vi "LC-MISDK_Meas_sub.vi"(0 ".NET refnum入力":refnum<k24>, 1 "Get Measurement Data":T1(radio)=enum."Lvxy", 8 "COM":i32) -> (10 "Duv":dbl, 12 "ReadLatestData Error":dbl format="%#_6f", 13 "Tcp":dbl, 14 "Lv 4":dbl, 15 "x":dbl, 16 "Z":dbl, 17 "Y":dbl, 18 "Lv 3":dbl, 19 "Dw":dbl, 20 "y":dbl, 21 "Lv":dbl, 22 "Pe":dbl, 23 "X":dbl, 24 "vd":dbl, 25 "Lv 2":dbl, 26 "ud":dbl)   [LabVIEW 2019]
uses:
  C:/Program Files (x86)/National Instruments/LabVIEW 2019/LC-MISDK.dll
  Program Files (x86)/National Instruments/LabVIEW 2019/LC-MISDK.dll
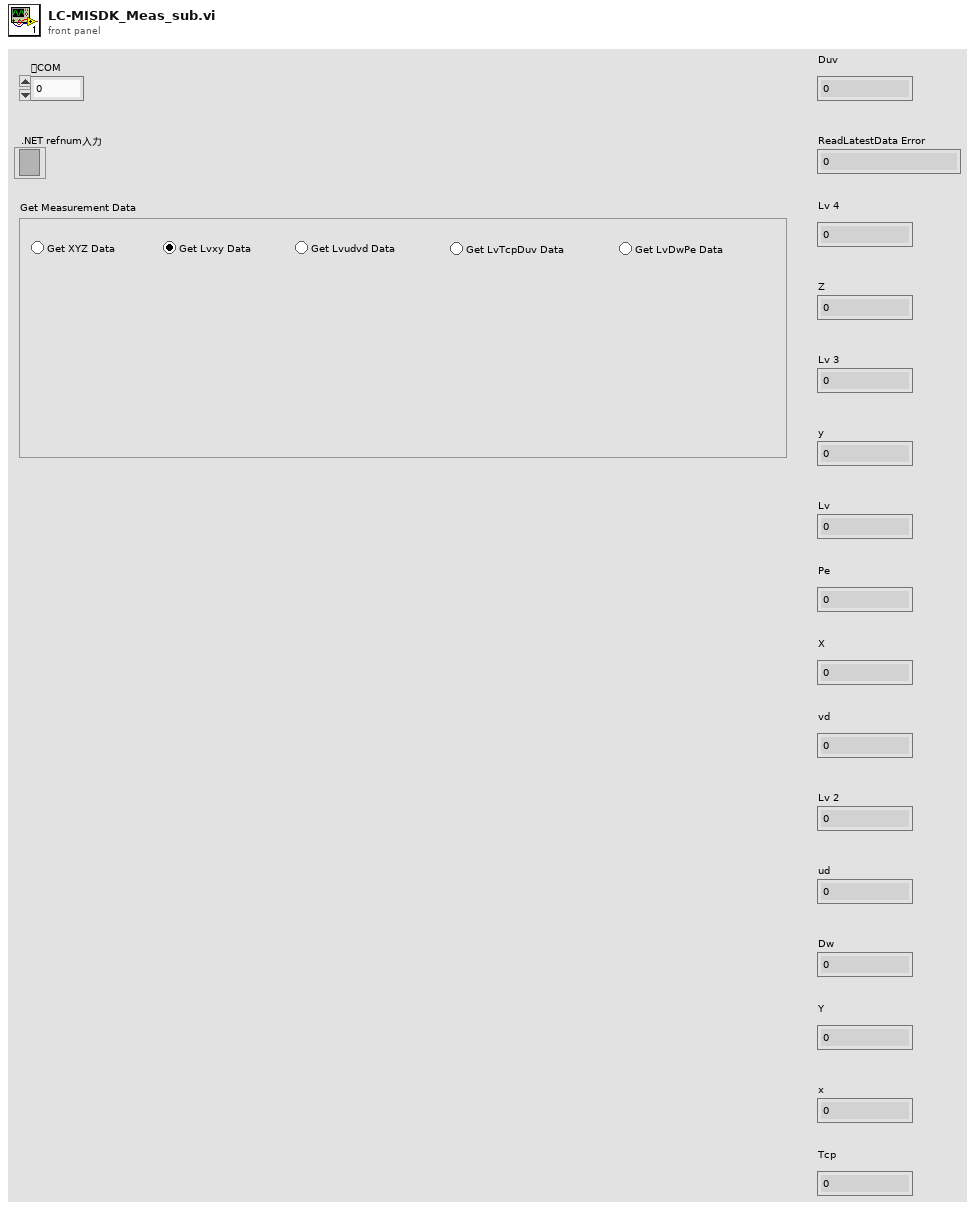
[diagram p1: front panel]
types:
  T1 = enum32{"XYZ", "Lvxy", "Lvudvd", "LvTcpDuv", "LvDwPe"}
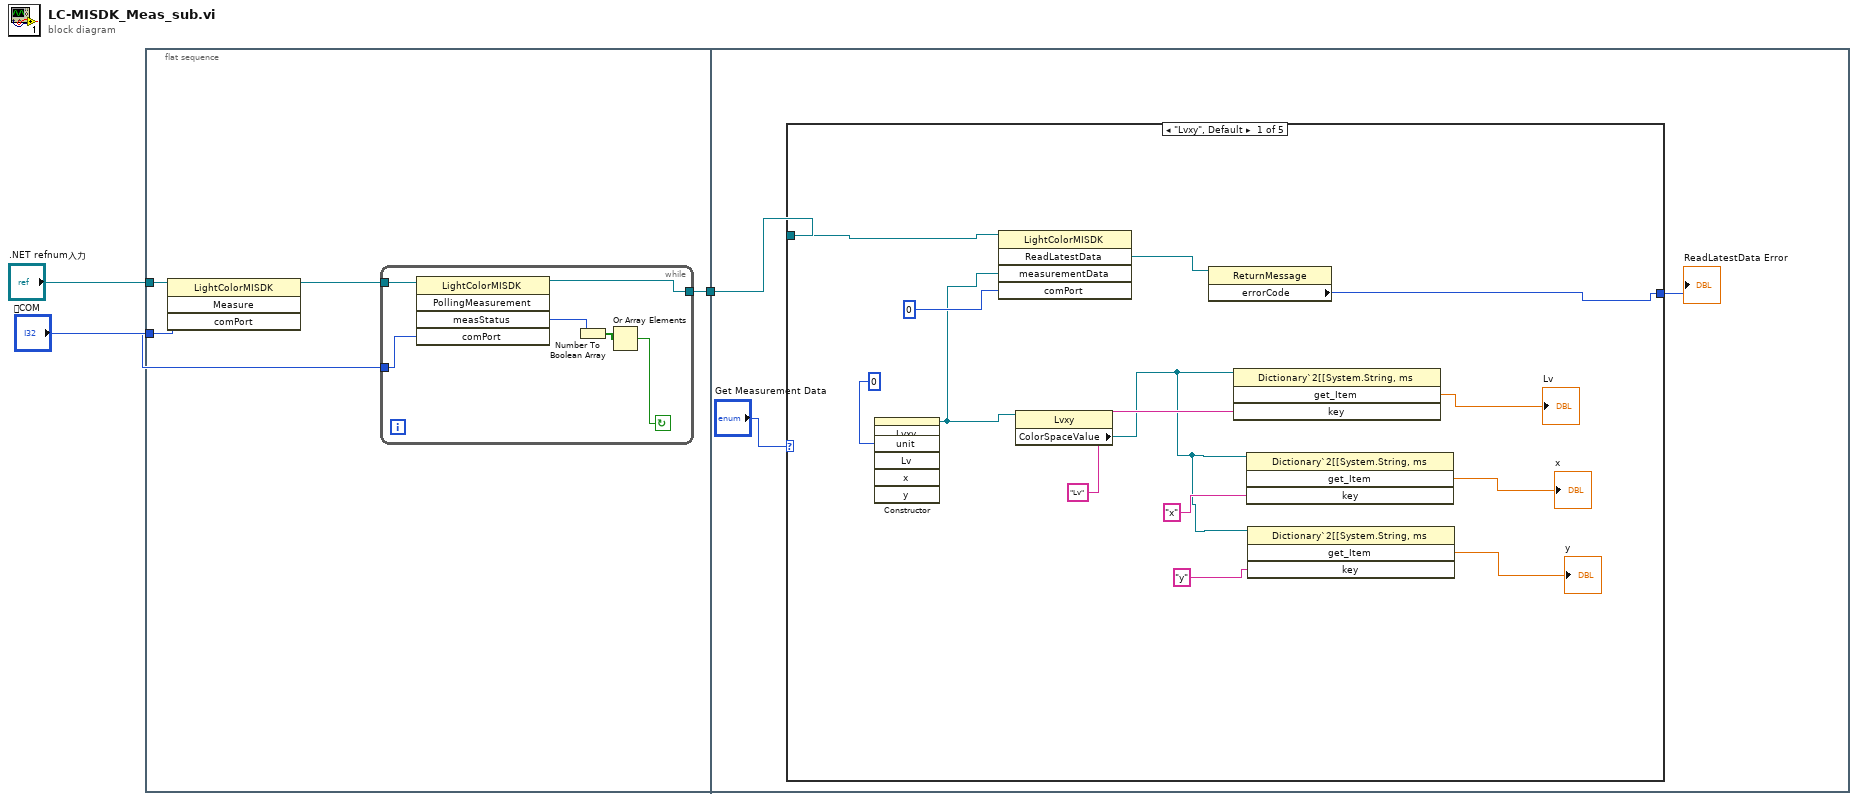
[diagram p0: block diagram]
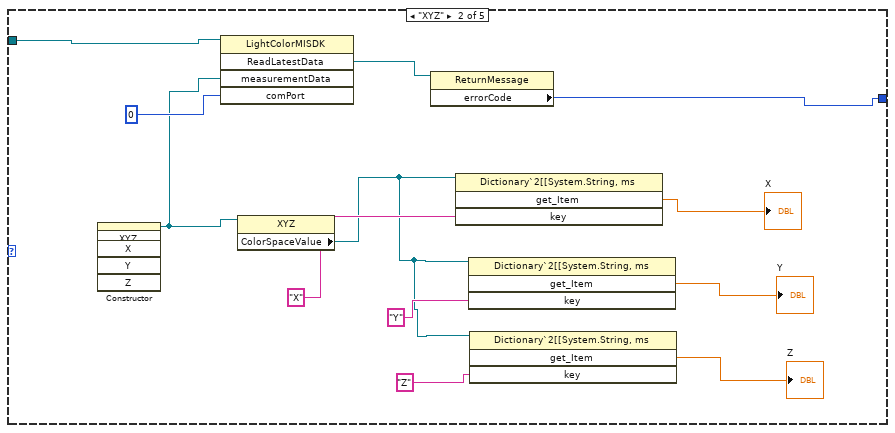
[diagram p2: hidden frame]
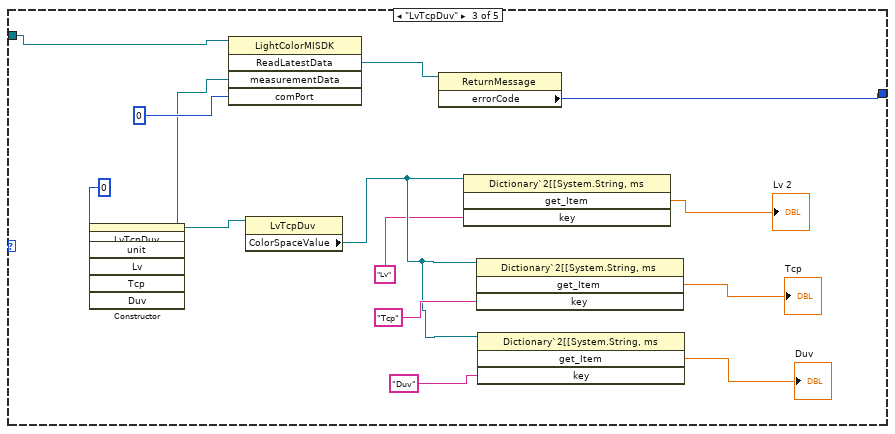
[diagram p3: hidden frame]
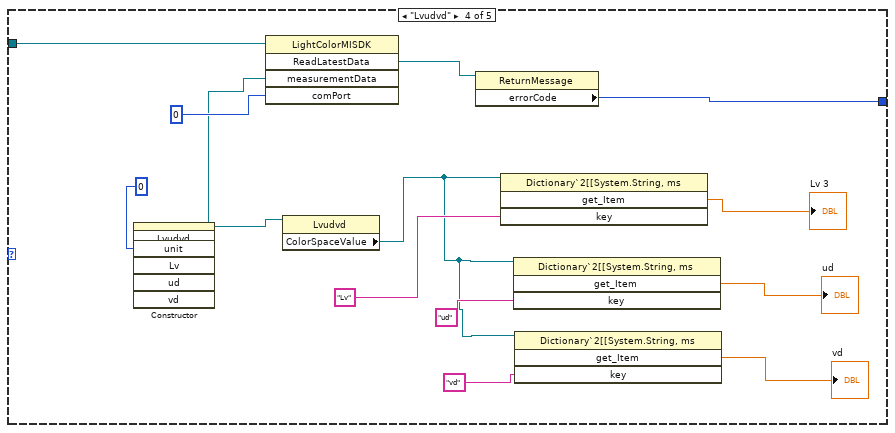
[diagram p4: hidden frame]
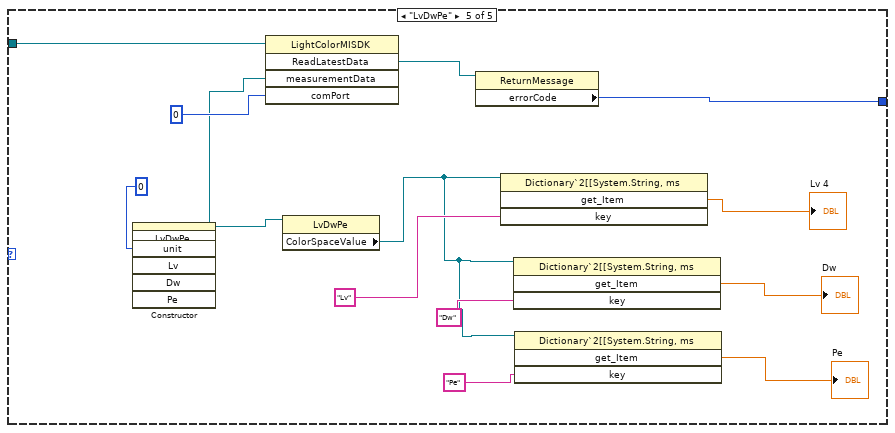
[diagram p5: hidden frame]
diagram:
  n1 = flat-sequence {
    tunnel: ".NET refnum入力" -> [w6]
    tunnel: "COM" -> [w4]
    tunnel: [w7] -> w3
    tunnel: w3 -> [w15]
    frame #0 {
      n2 = invoke on="インボークノード" class="LightColorMISDK" method="Measure"(reference=w6, "comPort"=w4) -> (reference out=w5:refnum<k24>)  [unwired: 2 in, 3 out]
      n3 = while {
        tunnel: [w12] -> w7
        tunnel: w5 -> [w11]
        tunnel: w4 -> [w10]
        stop <- w8 continue-if-true
        n4 = invoke on="インボークノード" class="LightColorMISDK" method="PollingMeasurement"(reference=w11, "comPort"=w10) -> (reference out=w12:refnum<k24>, "measStatus"=w13:i32)  [unwired: 3 in, 3 out]
        n5 = Number To Boolean Array(number=w13) -> (Boolean array=w9:bool[])
        n6 = Or Array Elements(Boolean array=w9) -> (logical OR=w8:bool)
      }
    }
    frame #1 {
      n7 = case shown="\"Lvxy\", Default" "Get Measurement Data" {
        tunnel: w15 -> [w29 w41 w54 w67 w80]
        tunnel: [w17 w30 w42 w55 w68] -> w14
        frame "Lvxy", Default {
          n8 = constructor class="Lvxy"("unit"=0) -> (reference out=w26:refnum<k24>)  [unwired: 6 in, 6 out]
          n9 = invoke on="インボークノード" class="LightColorMISDK" method="ReadLatestData"(reference=w29, "measurementData"=w26, "comPort"=0) -> ("ReadLatestData"=w27:refnum<k24>)  [unwired: 2 in, 4 out]
          n10 = property class="Lvxy"(reference=w26) -> ("ColorSpaceValue"=w21:refnum<k24>)  [unwired: 1 in, 2 out]
          n11 = property on="プロパティノード" class="ReturnMessage"(reference=w27) -> ("errorCode"=w17:i32)  [unwired: 1 in, 2 out]
          n12 = invoke class="Dictionary`2[[System.String, ms" method="get_Item"(reference=w21, "key"="Lv") -> ("get_Item"=→"Lv":dbl)  [unwired: 2 in, 3 out]
          n13 = invoke class="Dictionary`2[[System.String, ms" method="get_Item"(reference=w21, "key"="x") -> ("get_Item"=→"x":dbl)  [unwired: 2 in, 3 out]
          n14 = invoke class="Dictionary`2[[System.String, ms" method="get_Item"(reference=w21, "key"="y") -> ("get_Item"=→"y":dbl)  [unwired: 2 in, 3 out]
        }
        frame "XYZ" {
          n15 = constructor class="XYZ"() -> (reference out=w38:refnum<k24>)  [unwired: 6 in, 5 out]
          n16 = invoke on="インボークノード" class="LightColorMISDK" method="ReadLatestData"(reference=w41, "measurementData"=w38, "comPort"=0) -> ("ReadLatestData"=w39:refnum<k24>)  [unwired: 2 in, 4 out]
          n17 = property class="XYZ"(reference=w38) -> ("ColorSpaceValue"=w33:refnum<k24>)  [unwired: 1 in, 2 out]
          n18 = property on="プロパティノード" class="ReturnMessage"(reference=w39) -> ("errorCode"=w30:i32)  [unwired: 1 in, 2 out]
          n19 = invoke class="Dictionary`2[[System.String, ms" method="get_Item"(reference=w33, "key"="X") -> ("get_Item"=→"X":dbl)  [unwired: 2 in, 3 out]
          n20 = invoke class="Dictionary`2[[System.String, ms" method="get_Item"(reference=w33, "key"="Y") -> ("get_Item"=→"Y":dbl)  [unwired: 2 in, 3 out]
          n21 = invoke class="Dictionary`2[[System.String, ms" method="get_Item"(reference=w33, "key"="Z") -> ("get_Item"=→"Z":dbl)  [unwired: 2 in, 3 out]
        }
        frame "LvTcpDuv" {
          n22 = constructor class="LvTcpDuv"("unit"=0) -> (reference out=w51:refnum<k24>)  [unwired: 6 in, 6 out]
          n23 = invoke on="インボークノード" class="LightColorMISDK" method="ReadLatestData"(reference=w54, "measurementData"=w51, "comPort"=0) -> ("ReadLatestData"=w52:refnum<k24>)  [unwired: 2 in, 4 out]
          n24 = property class="LvTcpDuv"(reference=w51) -> ("ColorSpaceValue"=w47:refnum<k24>)  [unwired: 1 in, 2 out]
          n25 = property on="プロパティノード" class="ReturnMessage"(reference=w52) -> ("errorCode"=w42:i32)  [unwired: 1 in, 2 out]
          n26 = invoke class="Dictionary`2[[System.String, ms" method="get_Item"(reference=w47, "key"="Lv") -> ("get_Item"=→"Lv 2":dbl)  [unwired: 2 in, 3 out]
          n27 = invoke class="Dictionary`2[[System.String, ms" method="get_Item"(reference=w47, "key"="Tcp") -> ("get_Item"=→"Tcp":dbl)  [unwired: 2 in, 3 out]
          n28 = invoke class="Dictionary`2[[System.String, ms" method="get_Item"(reference=w47, "key"="Duv") -> ("get_Item"=→"Duv":dbl)  [unwired: 2 in, 3 out]
        }
        frame "Lvudvd" {
          n29 = constructor class="Lvudvd"("unit"=0) -> (reference out=w64:refnum<k24>)  [unwired: 6 in, 6 out]
          n30 = invoke on="インボークノード" class="LightColorMISDK" method="ReadLatestData"(reference=w67, "measurementData"=w64, "comPort"=0) -> ("ReadLatestData"=w65:refnum<k24>)  [unwired: 2 in, 4 out]
          n31 = property class="Lvudvd"(reference=w64) -> ("ColorSpaceValue"=w59:refnum<k24>)  [unwired: 1 in, 2 out]
          n32 = property on="プロパティノード" class="ReturnMessage"(reference=w65) -> ("errorCode"=w55:i32)  [unwired: 1 in, 2 out]
          n33 = invoke class="Dictionary`2[[System.String, ms" method="get_Item"(reference=w59, "key"="Lv") -> ("get_Item"=→"Lv 3":dbl)  [unwired: 2 in, 3 out]
          n34 = invoke class="Dictionary`2[[System.String, ms" method="get_Item"(reference=w59, "key"="ud") -> ("get_Item"=→"ud":dbl)  [unwired: 2 in, 3 out]
          n35 = invoke class="Dictionary`2[[System.String, ms" method="get_Item"(reference=w59, "key"="vd") -> ("get_Item"=→"vd":dbl)  [unwired: 2 in, 3 out]
        }
        frame "LvDwPe" {
          n36 = constructor class="LvDwPe"("unit"=0) -> (reference out=w77:refnum<k24>)  [unwired: 6 in, 6 out]
          n37 = invoke on="インボークノード" class="LightColorMISDK" method="ReadLatestData"(reference=w80, "measurementData"=w77, "comPort"=0) -> ("ReadLatestData"=w78:refnum<k24>)  [unwired: 2 in, 4 out]
          n38 = property class="LvDwPe"(reference=w77) -> ("ColorSpaceValue"=w72:refnum<k24>)  [unwired: 1 in, 2 out]
          n39 = property on="プロパティノード" class="ReturnMessage"(reference=w78) -> ("errorCode"=w68:i32)  [unwired: 1 in, 2 out]
          n40 = invoke class="Dictionary`2[[System.String, ms" method="get_Item"(reference=w72, "key"="Lv") -> ("get_Item"=→"Lv 4":dbl)  [unwired: 2 in, 3 out]
          n41 = invoke class="Dictionary`2[[System.String, ms" method="get_Item"(reference=w72, "key"="Dw") -> ("get_Item"=→"Dw":dbl)  [unwired: 2 in, 3 out]
          n42 = invoke class="Dictionary`2[[System.String, ms" method="get_Item"(reference=w72, "key"="Pe") -> ("get_Item"=→"Pe":dbl)  [unwired: 2 in, 3 out]
        }
      }
      "ReadLatestData Error" <- w14
    }
  }
